vi "随即温度.vi"() -> ()   [LabVIEW 2018]
panel:
  out "温度计":dbl(slide) scale=-100.0..100.0
  out "波形图表":dbl(graph)
  in  "停止":bool
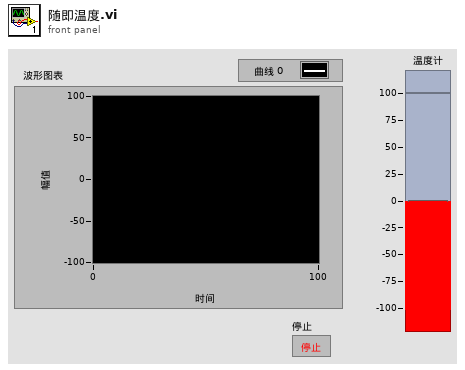
[diagram p1: front panel]
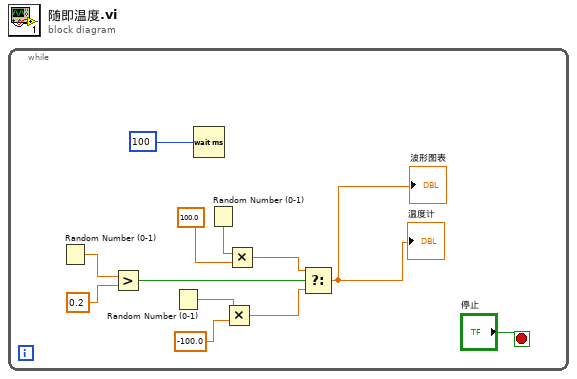
[diagram p0: block diagram]
diagram:
  n1 = while {
    stop <- "停止" stop-if-true
    n2 = Random Number (0-1)() -> (number: 0 to 1=w9:dbl)
    n3 = Greater?(x=w9, y=0.2) -> (0:w8:bool)
    n4 = Random Number (0-1)() -> (number: 0 to 1=w3:dbl)
    n5 = Wait (ms)(milliseconds to wait=u32 100 ("毫秒计时值")) -> ()  [unwired: 1 out]
    n6 = Random Number (0-1)() -> (number: 0 to 1=w6:dbl)
    n7 = Multiply(x=w3, y=-100.0) -> (x*y=w2:dbl)
    n8 = Multiply(x=w6, y=100.0) -> (x*y=w5:dbl)
    n9 = Select(t=w5, s=w8, f=w2) -> (s? t:f=→"波形图表" →"温度计":dbl)
  }
